vi "DropletFile_Headers_GCFS.vi"(2 "error in (no error)":errorcluster, 3 "path":path) -> (0 "error out":errorcluster, 1 "File path":path)   [LabVIEW 2024]
uses:
  <vilib>/Utility/file.llb/Write Delimited Spreadsheet (string).vi
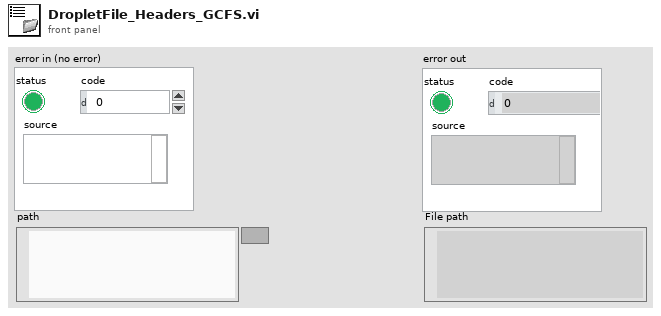
[diagram p1: front panel]
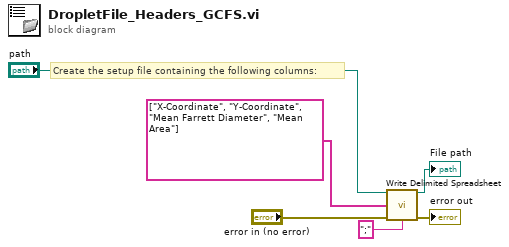
[diagram p0: block diagram]
diagram:
  # "Create the setup file containing the following columns:"
  n1 = call-poly <vilib>:"Write Delimited Spreadsheet.vi"("file path (dialog if empty)"="path", "1D data"=string[] ["X-Coordinate", "Y-Coordinate", "Mean Farrett Diameter", "Mean Area"], "error in (no error)"="error in (no error)", "delimiter (\\t)"=";" ("delimiter (\\t)")) -> ("new file path (Not A Path if cancelled)"=→"File path":path, "error out"=→"error out":errorcluster)  [unwired: 10 in]
